vi "TxtFile.vi"   [LabVIEW 2020]
panel:
  # "Write Txt File"
types:
  T1 = enum16{"open", "replace", "create", "open or create", "replace or create", "replace or create with confirmation"}
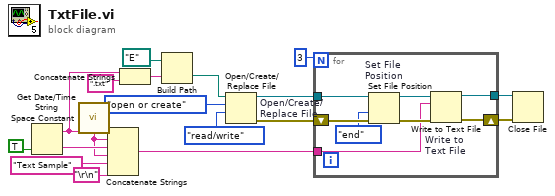
[diagram p0: block diagram]
diagram:
  n1 = Get Date/Time String(want seconds? (F)=TRUE) -> (date string=w14:string, time string=w13:string)  [unwired: 2 out]
  n2 = call <vilib>:"Space Constant.vi"() -> ("String"=w5:string)
  n3 = Concatenate Strings(w14, w5, w13, w5, "Text Sample" ("string"), "\r\n") -> (w4:string)
  n4 = Concatenate Strings(w14, ".txt" ("string")) -> (w16:string)
  n5 = Build Path(base path=path "E:/", name or relative path=w16) -> (appended path=w15:path)
  n6 = Open/Create/Replace File "Open/Create/\nReplace File"(file path (use dialog)=w15, operation (0:open)=T1."open or create", access (0:read/write)=enum16{"read/write", "read-only", "write-only"}."read/write") -> (refnum out=w9:refnum<file>, error out=w8:errorcluster)  [unwired: 1 in, 3 out]
  n7 = for {
    N: 3 -> [_]
    tunnel: [w26] -> w11
    tunnel: w9 -> [w24]
    tunnel: w4 -> [w19]
    shift-right: [w25] -> w10
    shift-left: w8 -> [w23]
    n8 = Set File Position "Set File\nPosition"(refnum=w24, from (0:start)=enum16{"start", "end", "current"}."end", error in=w23) -> (refnum out=w21:refnum<file>, error out=w20:errorcluster)  [unwired: 1 out]
    n9 = Write to Text File "Write to \nText File"(file (use dialog)=w21, text=w19, error in=w20) -> (refnum out=w26:refnum<file>, error out=w25:errorcluster)  [unwired: 2 out]
  }
  n10 = Close File(refnum=w11, error in=w10) -> ()  [unwired: 2 out]
